vi "wrap.PullNumber.vi"(0 "class.GLue in":refnum<class "class.GLue.lvclass">, 11 "error in (no error)":errorcluster, 13 "Index":i32=-1) -> (4 "class.GLue out":refnum<class "class.GLue.lvclass">, 8 "Number":dbl, 15 "error out":errorcluster)   [LabVIEW 2014, in "GLue.lvlib" / "class.GLue.lvclass"]
uses:
  class.GLue.lvclass
  class.GLue.lvclass/class.GLue.ctl
  Resources/GLue.dll
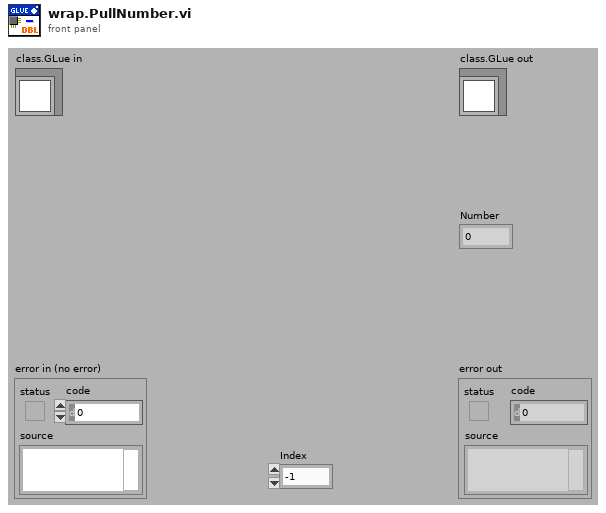
[diagram p1: front panel]
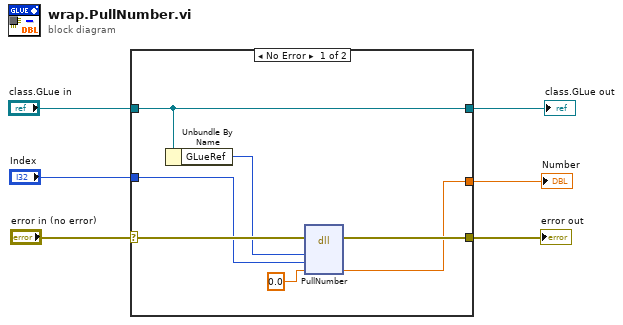
[diagram p0: block diagram]
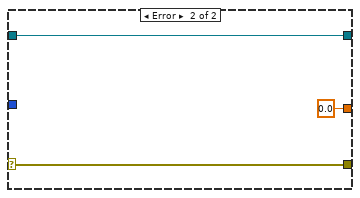
[diagram p2: hidden frame]
diagram:
  n1 = case shown="No Error" "error in (no error)" {
    selector: "error in (no error)" -> [w12 w16]
    tunnel: [w11 w16] -> w5
    tunnel: [w13 w15] -> w3
    tunnel: "class.GLue in" -> [w13 w15]
    tunnel: "Index" -> [w8 _]
    tunnel: [w7 0.0 ("Number")] -> w1
    frame No Error {
      n2 = Unbundle By Name(w13) -> ("GLueRef"=w10:i64)
      n3 = dll-call lib="C:/Users/Antonie/Documents/work/glue/trunk/Resources/GLue.dll" fn="PullNumber"(error in=w12, "MLua"=w10, "Index"=w8, "double"=0.0 ("Bool")) -> (error out=w11:errorcluster, "double"=w7:dbl)  [unwired: 5 in, 1 out]
    }
    frame Error {
    }
  }
  "error out" <- w5
  "class.GLue out" <- w3
  "Number" <- w1
